vi "IV-Tracer_v1.01.vi"() -> ()   [LabVIEW 2014]
doc: "Configures a sweep and takes voltage and current readings at each point."
uses:
  <instrlib>/Keithley 24XX/Public/Data/Read (Multiple Points).vi
  <instrlib>/Keithley 24XX/Keithley 24XX.lvlib
panel:
  out "Data IV Keithley":string
  in  "Data IV Keithley":path=path "C:/Users/Administrator/Documents/Device-characterization-setup/IV-Trace/Data/dumb/2015_xx_xx_xxxx_xx_keithley_001.txt"
  out "IV Curve":cluster{"Voltage":sgl[], "Current":sgl[]}(graph)
  out "Data Resistivity":string
  in  "Data Resistivity":path=path "C:/Users/Administrator/Documents/Device-characterization-setup/IV-Trace/Data/dumb/2015_xx_xx_xxxx_xx_keithley_resistivity_001.txt"
  out "Resistance-Voltage":cluster{sgl[], sgl[]}(graph)
  in  "Source Mode  (0: Voltage)":u16(ring) items=["Voltage", "Current"]
  in  "Serial Configuration":T1={"Baud Rate"=9600, "Parity"=0, "Data Bits"=8, "Stop Bits"=10, "Flow Control"=0} {"Flow Control" items=["None", "XON/XOFF", "RTS/CTS", "XON/XOFF & RTS/CTS", "DTR/DSR", "XON/XOFF & DTR/DSR"]; "Stop Bits" items=["1.0"=10, "1.5"=15, "2.0"=20]; "Data Bits" items=["7"=7, "8"=8]; "Parity" items=["None", "Odd", "Even", "Mark", "Space"]; "Baud Rate" items=["300"=300, "600"=600, "1200"=1200, "2400"=2400, "4800"=4800, "9600"=9600, "19200"=19200]}
  in  "VISA resource name":refnum<visa-resource-name>="GPIB9::24::INSTR"
  in  "Timeout (10000 ms)":i32=10000 format="%#.6g"
  in  "Maximum Amplitude (2)":dbl=2.0
  in  "Minimum Amplitude (1)":dbl=1.0
  in  "Number of Points (5)":u32=5
  in  "Compliance  Level (1)":dbl=1.0
  # "NanoBEEs 2015-IV Tracer v1.01"
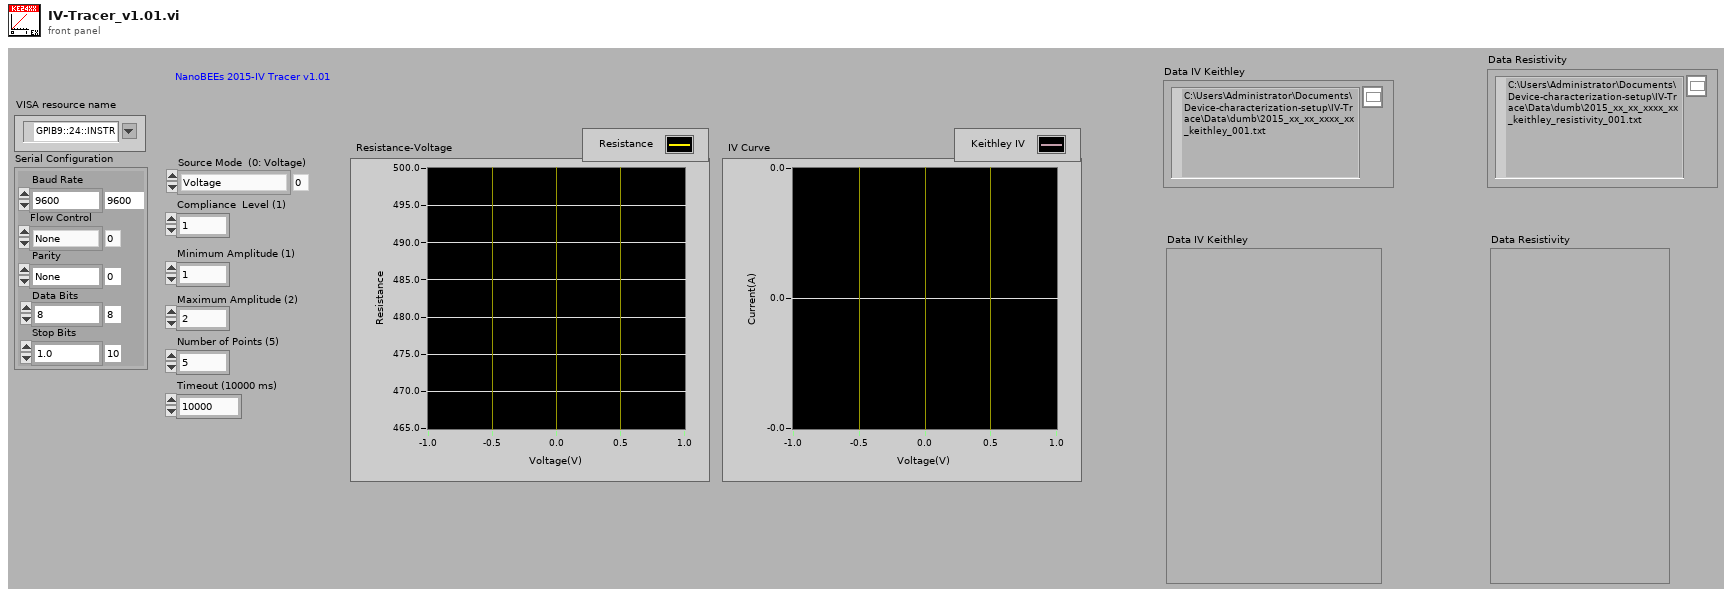
[diagram p1: front panel]
types:
  T1 = cluster{"Baud Rate":u32, "Parity":u16, "Data Bits":u16, "Stop Bits":u16, "Flow Control":u16}
  T2 = enum16{"open", "replace", "create", "open or create", "replace or create", "replace or create with confirmation"}
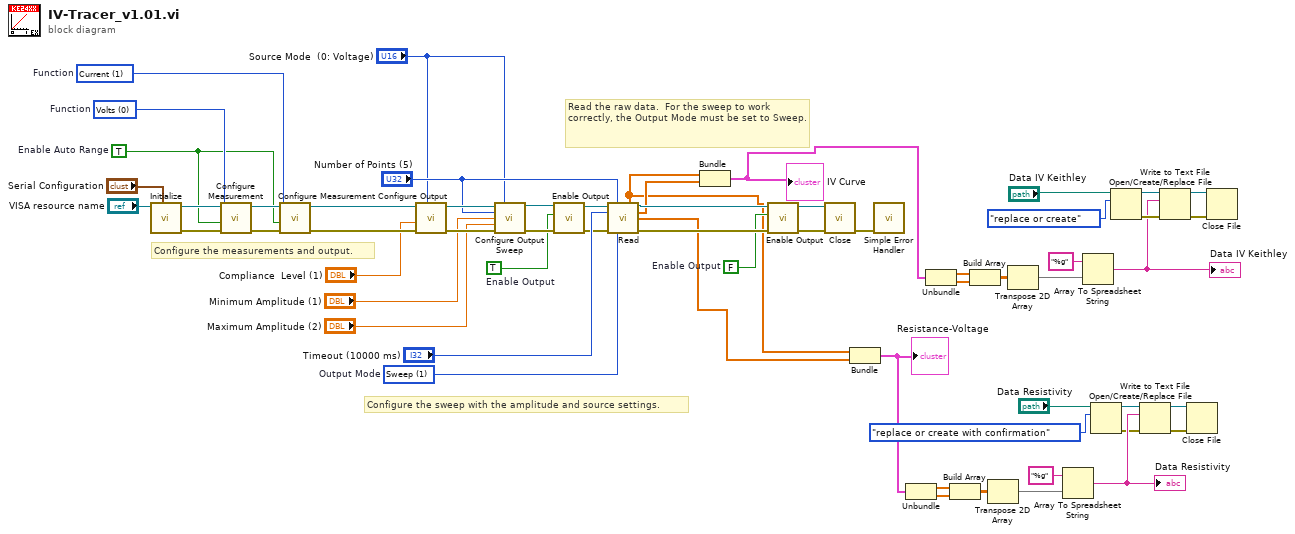
[diagram p0: block diagram]
diagram:
  w31 = TRUE  # Enable Output
  w32 = TRUE  # Enable Auto Range
  w33 = u16 1 items=["Volts", "Current", "Resistance"]  # Function
  w34 = u16 0 items=["Volts", "Current", "Resistance"]  # Function
  w40 = FALSE  # Enable Output
  w46 = u16 1 items=["Fixed", "Sweep", "List"]  # Output Mode
  # "Read the raw data.  For the sweep to work correctly, the Output Mode must be set to Sweep."
  # "Configure the sweep with the amplitude and source settings."
  # "Configure the measurements and output."
  n1 = call <instrlib>:"Initialize.vi"("Serial Configuration"="Serial Configuration", "VISA resource name"="VISA resource name") -> ("error out"=w59:errorcluster, "VISA resource name out"=w60:refnum<visa-resource-name>)  [unwired: 8 in]
  n2 = call <instrlib>:"Configure Measurement.vi"("error in (no error)"=w59, "Enable Auto Range (T:Enable)"=w32, "Function (0: Volts)"=w34, "VISA resource name"=w60) -> ("error out"=w58:errorcluster, "VISA resource name out"=w57:refnum<visa-resource-name>)  [unwired: 6 in]
  n3 = call <instrlib>:"Configure Measurement.vi"("error in (no error)"=w58, "Enable Auto Range (T:Enable)"=w32, "Function (0: Volts)"=w33, "VISA resource name"=w57) -> ("error out"=w55:errorcluster, "VISA resource name out"=w56:refnum<visa-resource-name>)  [unwired: 6 in]
  n4 = call <instrlib>:"Configure Output.vi"("Source Mode  (0: Voltage)"="Source Mode  (0: Voltage)", "error in (no error)"=w55, "Compliance  Level (0.1)"="Compliance  Level (1)", "VISA resource name"=w56) -> ("error out"=w54:errorcluster, "VISA resource name out"=w53:refnum<visa-resource-name>)  [unwired: 6 in]
  n5 = call <instrlib>:"Configure Output Sweep.vi"("VISA resource name"=w53, "Source Mode  (0: Voltage)"="Source Mode  (0: Voltage)", "Number of Points (5)"="Number of Points (5)", "Minimum Amplitude (1)"="Minimum Amplitude (1)", "Maximum Amplitude (2)"="Maximum Amplitude (2)", "error in (no error)"=w54) -> ("VISA resource name out"=w37:refnum<visa-resource-name>, "error out"=w36:errorcluster)  [unwired: 8 in]
  n6 = call <instrlib>:"Enable Output.vi"("error in (no error)"=w36, "Enable Output (T: Enable)"=w31, "VISA resource name"=w37) -> ("error out"=w39:errorcluster, "VISA resource name out"=w38:refnum<visa-resource-name>)  [unwired: 7 in]
  n7 = call-poly <instrlib>:"Read.vi"("VISA resource name"=w38, "Sample Count (1)"="Number of Points (5)", "Timeout (10000 ms)"="Timeout (10000 ms)", "error in (no error)"=w39, "Output Mode (0: Fixed)"=w46) -> ("Voltage"=w4:sgl[], "VISA resource name out"=w41:refnum<visa-resource-name>, "Current"=w29:sgl[], "Resistance"=w5:sgl[], "error out"=w42:errorcluster)  [unwired: 4 in, 2 out]
  n8 = Bundle("Voltage"=w4, "Current"=w29) -> (w3:cluster{"Voltage":sgl[], "Current":sgl[]})  [unwired: 1 out]
  "IV Curve" <- w3
  n9 = call <instrlib>:"Enable Output.vi"("error in (no error)"=w42, "Enable Output (T: Enable)"=w40, "VISA resource name"=w41) -> ("error out"=w43:errorcluster, "VISA resource name out"=w44:refnum<visa-resource-name>)  [unwired: 7 in]
  n10 = call <instrlib>:"Close.vi"("error in (no error)"=w43, "VISA resource name"=w44) -> ("error out"=w45:errorcluster)  [unwired: 9 in]
  n11 = Bundle("Voltage"=w4, "Resistance"=w5) -> (w12:cluster{"Voltage":sgl[], "Resistance":sgl[]})  [unwired: 1 out]
  "Resistance-Voltage" <- w12
  n12 = call <vilib>:"Simple Error Handler.vi"("error in (no error)"=w45) -> ()  [unwired: 4 in, 5 out]
  n13 = Unbundle(w12) -> ("Voltage"=w13:sgl[], "Resistance"=w14:sgl[])
  n14 = Unbundle(w3) -> ("Voltage"=w24:sgl[], "Current"=w25:sgl[])
  n15 = Build Array(w13, w14) -> (w15:sgl[][])
  n16 = Build Array(w24, w25) -> (w26:sgl[][])
  n17 = Transpose 2D Array(2D array=w15) -> (transposed array=w17:sgl[][])
  n18 = Transpose 2D Array(2D array=w26) -> (transposed array=w28:sgl[][])
  n19 = Array To Spreadsheet String(array=w17, 3:"%g" ("format string")) -> (spreadsheet string=w18:string)  [unwired: 1 in]
  "Data Resistivity" <- w18
  n20 = Array To Spreadsheet String(array=w28, 3:"%g" ("format string")) -> (spreadsheet string=w1:string)  [unwired: 1 in]
  "Data IV Keithley" <- w1
  n21 = Open/Create/Replace File(file path (use dialog)="Data Resistivity", operation (0:open)=T2."replace or create with confirmation") -> (refnum out=w11:refnum<file>, error out=w6:errorcluster)  [unwired: 4 in, 1 out]
  n22 = Open/Create/Replace File(file path (use dialog)="Data IV Keithley", operation (0:open)=T2."replace or create") -> (refnum out=w23:refnum<file>, error out=w19:errorcluster)  [unwired: 4 in, 1 out]
  n23 = Write to Text File(file (use dialog)=w11, text=w18, error in=w6) -> (refnum out=w8:refnum<file>, error out=w7:errorcluster)  [unwired: 2 out]
  n24 = Write to Text File(file (use dialog)=w23, text=w1, error in=w19) -> (refnum out=w21:refnum<file>, error out=w20:errorcluster)  [unwired: 2 out]
  n25 = Close File(refnum=w8, error in=w7) -> ()  [unwired: 2 out]
  n26 = Close File(refnum=w21, error in=w20) -> ()  [unwired: 2 out]
